vi "autonomus darrion style.vi"() -> ()   [LabVIEW 2010, in "Rampage.lvrbt"]
uses:
  Rampage.lvrbt
  <vilib>/NXT/Subs/MotorOutput.ctl
  <vilib>/NXT/NXTIO Xnodes/AddressXNode/NXTIOAddress.xnode
  <vilib>/NXT/Subs/MotorXNode.DC Motor Type.ctl
  <vilib>/NXT/Subs/MotorXNode.2DCMotor.ctl
  <vilib>/NXT/HiTechnic/HiTechnic Controls/HiTechnic Port.ctl
  <vilib>/NXT/Block Support/NXT_InputPort.ctl
  <vilib>/NXT/Subs/LVHSConnector.ctl
  <vilib>/NXT/NXTIO Xnodes/NXTIOXNode/NXTIO.xnode
  <vilib>/NXT/Subs/MotorXNode.1DCMotor.ctl
  <vilib>/NXT/Dual Mode Library/Waits/Wait_Num(msec).vi
  <vilib>/NXT/Dual Mode Library/prims/inRangeAndCoerce/inRangeAndCoerce_int.vi
  <vilib>/NXT/Dual Mode Library/Motors/MotorOn.vi
  <vilib>/NXT/Dual Mode Library/Waits/Wait_Num.vi
  <vilib>/NXT/NXTIO Xnodes/NXTIONodeSubVIs/TETRIX IO Move DC Motors.vi
  <vilib>/NXT/NXTIO Xnodes/NXTIONodeSubVIs/TETRIX IO Stop DC Motors.vi
  <vilib>/NXT/Dual Mode Library/Sensors/Light_On.vi
panel:
  in  "Centered Value":i16
  in  "Gain":i16
  in  "Base Speed":i16
  out "Enabled":bool
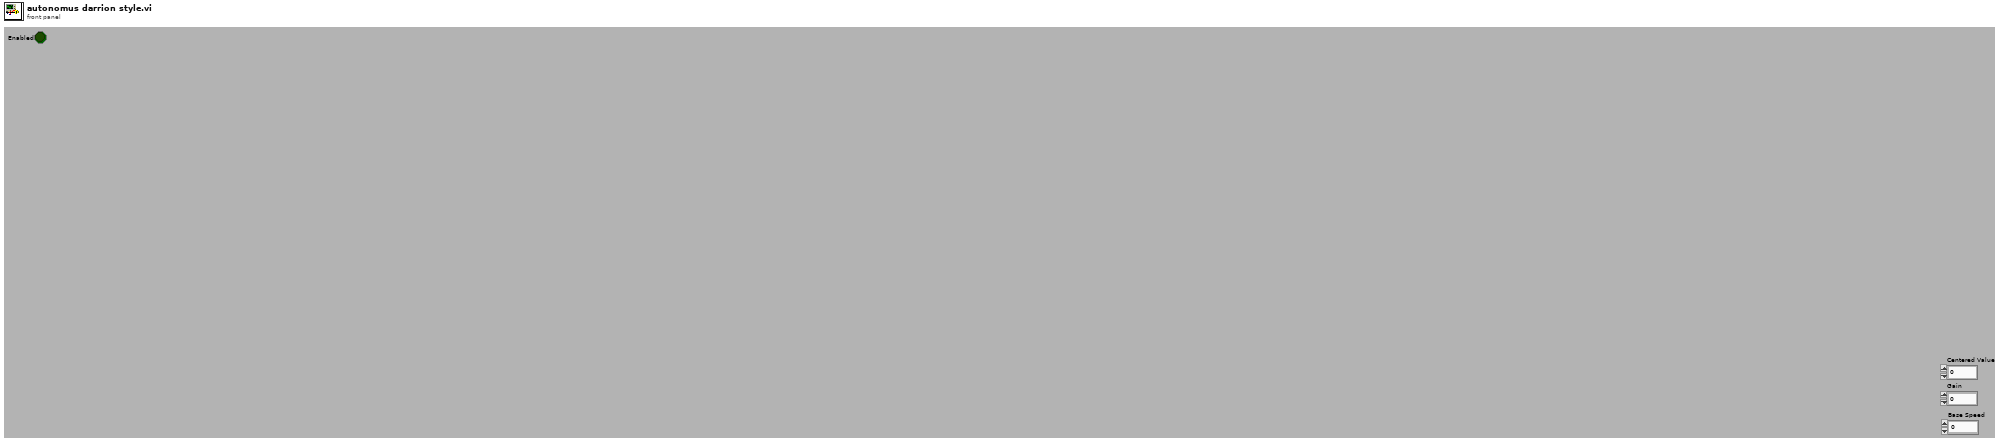
[diagram p1: front panel]
types:
  T1 = typedef "LVHSConnector.ctl" = cluster{"Hardware":string, "Flattened String":string}
  T2 = typedef "MotorOutput.ctl" = u8
  T3 = typedef "MotorXNode.DC Motor Type.ctl" = enum16{"DC Motor"}
  T4 = cluster{"DC Motor":T3, "Address":i16, "Address":i16}
  T5 = typedef "HiTechnic Port.ctl" = cluster{"Port":T6, "MUX Port":u8}
  T6 = typedef "NXT_InputPort.ctl" = u8
  T7 = cluster{"Direction (0-9)":i16, "Signal Strength (Array)":u8[]}
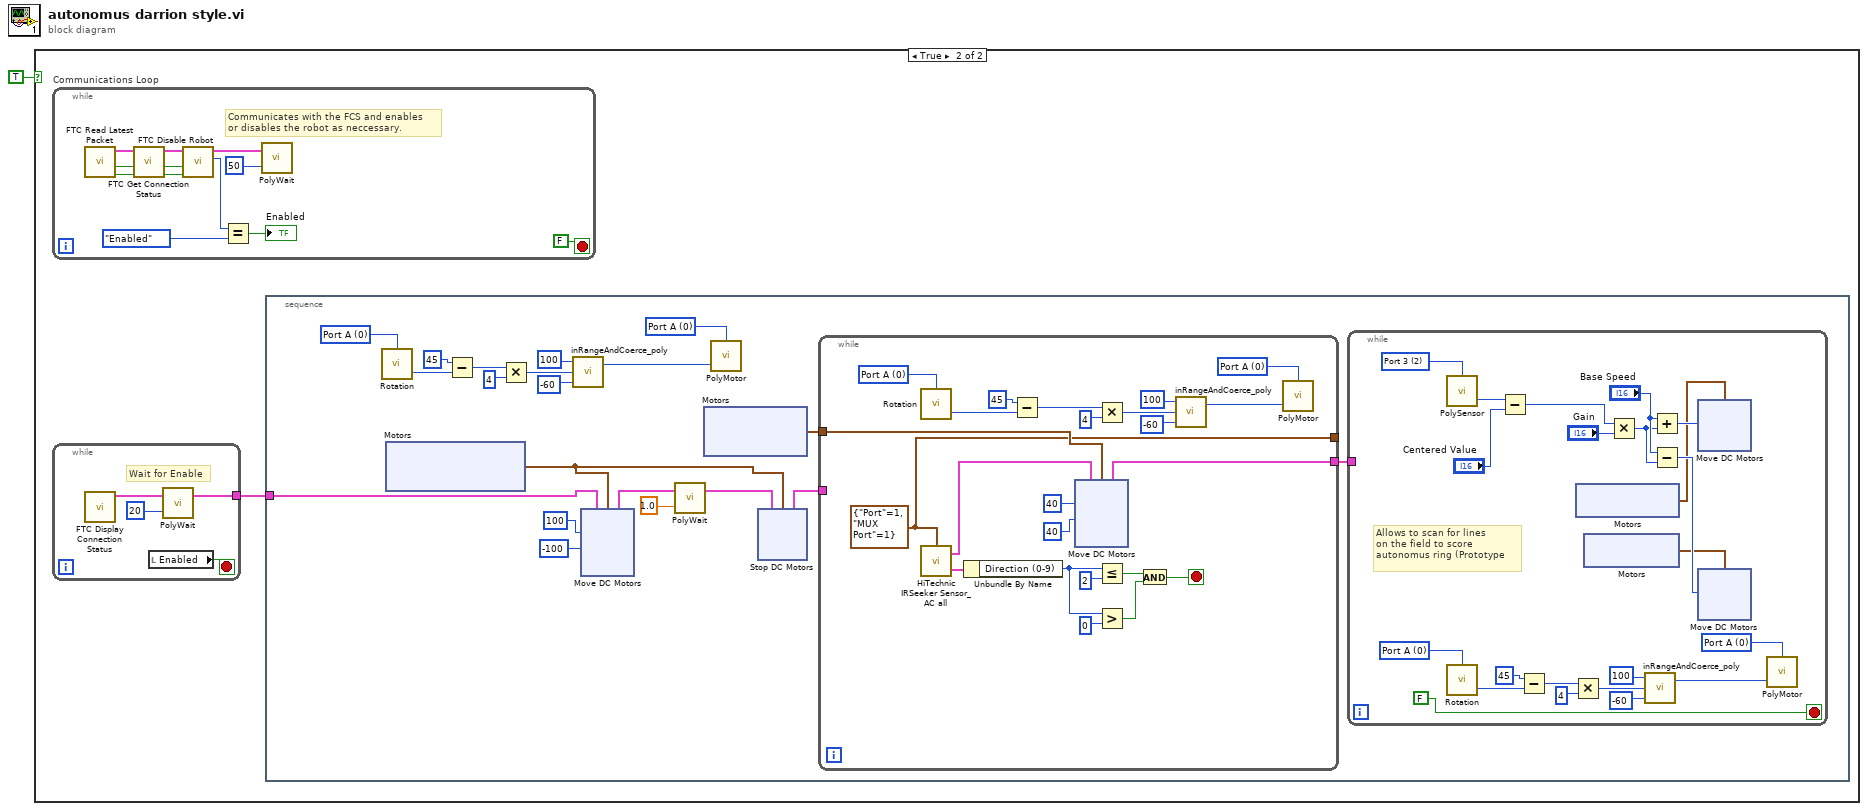
[diagram p0: block diagram]
diagram:
  n1 = case shown="True" TRUE {
    frame False {
    }
    frame True {
      n2 = while "Communications Loop" {
        stop <- FALSE stop-if-true
        # "Communicates with the FCS and enables \nor disables the robot as neccessary."
        n3 = call <vilib>:"FTC Read Latest Packet.vi"() -> ("Packet Received?"=w128:bool, "Stopped?"=w127:bool, "NXT"=w130:T1)  [unwired: 6 in, 3 out]
        n4 = call <vilib>:"FTC Get Connection Status.vi"("Packet Received?"=w128, "Stopped?"=w127, "NXT"=w130) -> ("Online?"=w119:bool, "Stopped?"=w120:bool, "NXT"=w129:T1)  [unwired: 5 in]
        n5 = call <vilib>:"FTC Disable Robot.vi"("Online?"=w119, "Stopped?"=w120, "NXT"=w129) -> ("Enabled?"=w123:enum16{"Disabled", "Enabled"}, "NXT"=w125:T1)  [unwired: 3 in]
        n6 = Equal?(x=w123, y=enum16{"Disabled", "Enabled"}."Enabled") -> (x = y?=→"Enabled":bool)
        n7 = call-poly <vilib>:"PolyWait.vi"("Time (100 msec)"=u32 50 ("Time (msec)"), "NXT"=w125) -> ()  [unwired: 2 in, 1 out]
      }
      n8 = while {
        tunnel: [w116] -> w2
        stop <- w117 stop-if-true
        # "Wait for Enable"
        n9 = call <vilib>:"FTC Display Connection Status.vi"() -> ("NXT"=w115:T1)  [unwired: 11 in]
        n10 = local read "Enabled"() -> (w117:bool)
        n11 = call-poly <vilib>:"PolyWait.vi"("Time (100 msec)"=u32 20 ("Time (msec)"), "NXT"=w115) -> ("NXT"=w116:T1)  [unwired: 2 in]
      }
      n12 = stacked-sequence {
        tunnel: w2 -> [w4]
        frame #0 {
          w14 = T2 0 items=["Port A"=0, "Port B"=1, "Port C"=2, "Ports A & B"=4, "Ports A & C"=5, "Ports B & C"=6, "All Ports"=3] ("Output Port (All Ports)")
          w12 = u8 0 items=["Port A", "Port B", "Port C"] ("Port (Port A)")
          n13 = call <vilib>:"Rotation.vi"("Port (Port A)"=w12) -> ("Angle of Rotation"=w15:i32)  [unwired: 2 in, 1 out]
          n14 = xnode "Motors"() -> ("DC Motor"=w22:T4)
          n15 = Subtract(x=45 ("Claw\nPosition"), y=w15) -> (x-y=w13:i32)
          n16 = Multiply(x=w13, y=4) -> (x*y=w11:i32)
          n17 = call-poly <vilib>:"inRangeAndCoerce_poly.vi"("lower limit"=-60, "x"=w11, "upper limit"=100) -> ("coerced(x)"=w8:i32)  [unwired: 1 out]
          n18 = xnode "Move DC Motors"("Power/Speed 1"=i8 100, "Motors"=w22, "NXT"=w4, "Power/Speed 2"=i8 -100) -> ("NXT"=w20:T1)
          n19 = call-poly <vilib>:"PolyWait.vi"("Time (1 sec)"=sgl 1.0, "NXT"=w20) -> ("NXT"=w17:T1)  [unwired: 2 in]
          n20 = xnode "Motors"() -> ("DC Motor"=w6:T4)
          n21 = call-poly <vilib>:"PolyMotor.vi"("Power (75)"=w8, "Output Port (All Ports)"=w14) -> ()  [unwired: 2 in, 1 out]
          n22 = xnode "Stop DC Motors"("Motors"=w22, "NXT"=w17) -> ("NXT"=w5:T1)
          n23 = while {
            tunnel: [w103] -> w3
            tunnel: w6 -> [w100]
            tunnel: [w87] -> _
            tunnel: w5 -> [_]
            stop <- w82 stop-if-true
            w92 = T2 0 items=["Port A"=0, "Port B"=1, "Port C"=2, "Ports A & B"=4, "Ports A & C"=5, "Ports B & C"=6, "All Ports"=3] ("Output Port (All Ports)")
            w94 = u8 0 items=["Port A", "Port B", "Port C"] ("Port (Port A)")
            w87 = T5 {"Port"=1, "MUX Port"=1} ("Port/MUX")
            n24 = call <vilib>:"Rotation.vi"("Port (Port A)"=w94) -> ("Angle of Rotation"=w91:i32)  [unwired: 2 in, 1 out]
            n25 = call <vilib>:"HiTechnic IRSeeker Sensor_AC all.vi"("Port/MUX"=w87) -> ("All Info"=w88:T7, "NXT"=w104:T1)  [unwired: 2 in]
            n26 = Unbundle By Name(w88) -> ("Direction (0-9)"=w85:i16)
            n27 = Subtract(x=45 ("Claw\nPosition"), y=w91) -> (x-y=w93:i32)
            n28 = xnode "Move DC Motors"("Power/Speed 2"=i8 40, "Power/Speed 1"=i8 40, "Motors"=w100, "NXT"=w104) -> ("NXT"=w103:T1)
            n29 = Multiply(x=w93, y=4) -> (x*y=w95:i32)
            n30 = Less Or Equal?(x=w85, y=i16 2) -> (x <= y?=w84:bool)
            n31 = Greater?(x=w85, y=i16 0) -> (0:w83:bool)
            n32 = And(x=w84, y=w83) -> (x .and. y?=w82:bool)
            n33 = call-poly <vilib>:"inRangeAndCoerce_poly.vi"("lower limit"=-60, "x"=w95, "upper limit"=100) -> ("coerced(x)"=w98:i32)  [unwired: 1 out]
            n34 = call-poly <vilib>:"PolyMotor.vi"("Power (75)"=w98, "Output Port (All Ports)"=w92) -> ()  [unwired: 2 in, 1 out]
          }
          n35 = while {
            tunnel: w3 -> [_]
            stop <- FALSE stop-if-true
            w30 = T2 0 items=["Port A"=0, "Port B"=1, "Port C"=2, "Ports A & B"=4, "Ports A & C"=5, "Ports B & C"=6, "All Ports"=3] ("Output Port (All Ports)")
            w28 = u8 0 items=["Port A", "Port B", "Port C"] ("Port (Port A)")
            w37 = T6 2 items=["Port 1", "Port 2", "Port 3", "Port 4"] ("Port (Port 3)")
            # "Allows to scan for lines\non the field to score \nautonomus ring (Prototype"
            n36 = call-poly <vilib>:"PolySensor.vi"("Port (Port 3)"=w37) -> ("Scaled Value"=w43:i16)  [unwired: 2 in, 1 out]
            n37 = call <vilib>:"Rotation.vi"("Port (Port A)"=w28) -> ("Angle of Rotation"=w31:i32)  [unwired: 2 in, 1 out]
            n38 = Subtract(x=w43, y="Centered Value") -> (x-y=w41:i16)
            n39 = Subtract(x=45 ("Claw\nPosition"), y=w31) -> (x-y=w29:i32)
            n40 = Multiply(x=w29, y=4) -> (x*y=w27:i32)
            n41 = xnode "Motors"() -> ("DC Motor"=w33:cluster{"DC Motor":T3, "Address":i16})
            n42 = xnode "Motors"() -> ("DC Motor"=w35:cluster{"DC Motor":T3, "Address":i16})
            n43 = Multiply(x=w41, y="Gain") -> (x*y=w34:i16)
            n44 = call-poly <vilib>:"inRangeAndCoerce_poly.vi"("lower limit"=-60, "x"=w27, "upper limit"=100) -> ("coerced(x)"=w24:i32)  [unwired: 1 out]
            n45 = Add(x="Base Speed", y=w34) -> (x+y=w38:i16)
            n46 = Subtract(x="Base Speed", y=w34) -> (x-y=w39:i16)
            n47 = xnode "Move DC Motors"("Power/Speed 1"=w38, "Motors"=w33) -> ()  [unwired: 1 in, 1 out]
            n48 = xnode "Move DC Motors"("Power/Speed 1"=w39, "Motors"=w35) -> ()  [unwired: 1 in, 1 out]
            n49 = call-poly <vilib>:"PolyMotor.vi"("Power (75)"=w24, "Output Port (All Ports)"=w30) -> ()  [unwired: 2 in, 1 out]
          }
        }
      }
    }
  }
